vi "StrafeScaling.vi"(0 "Raw Joystick Y":dbl, 5 "Raw Joystick X":dbl, 11 "Strafe Scaling":dbl(slide)=2.0 min=1.0 max=4.0 scale=1.0..4.0, 12 "joystickYInDeadband":bool, 13 "joystickXInDeadband":bool) -> (8 "Scaled Joystick Y":dbl, 15 "Scaled Joystick X":dbl)   [LabVIEW 2020]
doc: "Applies a deadband and nonlinear scaling to the strafe axes of a swerve drive. Includes a hook to override the non-linear deadband and scaling when the rotation is under autonomous control."
panel:
  in  "minimum":dbl=0.1
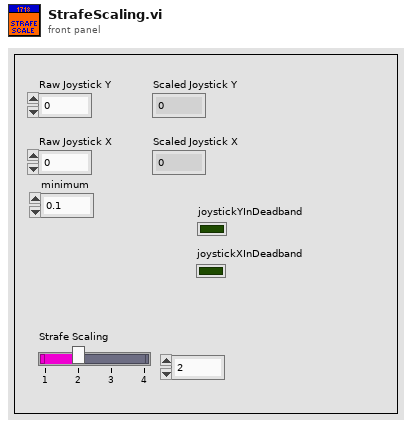
[diagram p1: front panel]
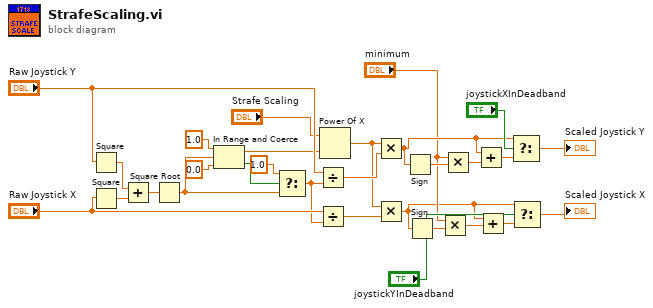
[diagram p0: block diagram]
diagram:
  n1 = Square(x="Raw Joystick Y") -> (x^2=w28:dbl)
  n2 = Square(x="Raw Joystick X") -> (x^2=w27:dbl)
  n3 = Add(x=w28, y=w27) -> (x+y=w29:dbl)
  n4 = Square Root(x=w29) -> (sqrt(x)=w22:dbl)
  n5 = In Range and Coerce(upper limit=1.0, x=w22, lower limit=0.0 ("upper limit")) -> (coerced(x)=w14:dbl, In Range?=w24:bool)
  n6 = Select(t=1.0, s=w24, f=w22) -> (s? t:f=w17:dbl)
  n7 = Divide(x="Raw Joystick Y", y=w17) -> (x/y=w21:dbl)
  n8 = Divide(x="Raw Joystick X", y=w17) -> (x/y=w18:dbl)
  n9 = Power Of X(1:w14, 2:"Strafe Scaling") -> (0:w15:dbl)
  n10 = Multiply(x=w15, y=w21) -> (x*y=w8:dbl)
  n11 = Multiply(x=w15, y=w18) -> (x*y=w2:dbl)
  n12 = Sign(1:w8) -> (0:w9:dbl)
  n13 = Sign(1:w2) -> (0:w5:dbl)
  n14 = Multiply(x="minimum", y=w5) -> (x*y=w3:dbl)
  n15 = Multiply(x="minimum", y=w9) -> (x*y=w10:dbl)
  n16 = Add(x=w8, y=w10) -> (x+y=w11:dbl)
  n17 = Add(x=w2, y=w3) -> (x+y=w4:dbl)
  n18 = Select(t=w8, s="joystickXInDeadband", f=w11) -> (s? t:f=→"Scaled Joystick Y":dbl)
  n19 = Select(t=w2, s="joystickYInDeadband", f=w4) -> (s? t:f=→"Scaled Joystick X":dbl)
